vi "Read C.vi"(8 "error in (no error)":errorcluster, 11 "Arithemetic Operation in":refnum<class "Arithemetic Operation.lvclass">) -> (0 "error out":errorcluster, 2 "C":dbl, 3 "Arithemetic Operation out":refnum<class "Arithemetic Operation.lvclass">)   [LabVIEW 2023, in "Arithemetic Operation.lvclass"]
uses:
  Arithemetic Operation.lvclass
  Arithemetic Operation.lvclass/Arithemetic Operation.ctl
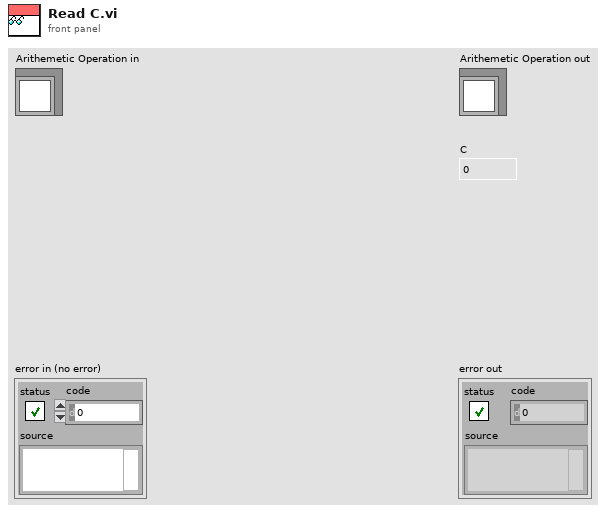
[diagram p1: front panel]
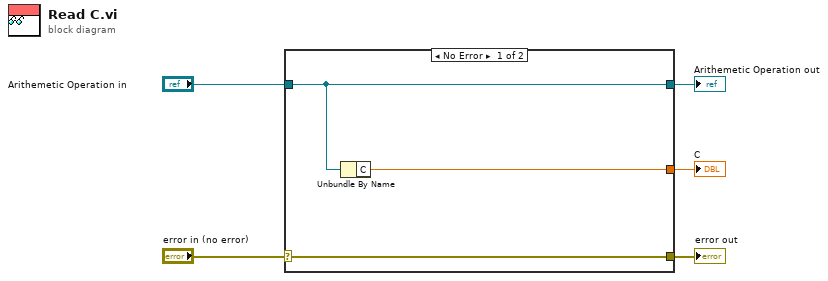
[diagram p0: block diagram]
diagram:
  n1 = case shown="No Error" "error in (no error)" {
    selector: "error in (no error)" -> [w8 w9]
    tunnel: [w8 w9] -> w4
    tunnel: [w7 w10] -> w2
    tunnel: "Arithemetic Operation in" -> [w7 w10]
    tunnel: [w6 _] -> w1
    frame No Error {
      n2 = Unbundle By Name(w7) -> ("C"=w6:dbl)
    }
    frame Error {
    }
  }
  "error out" <- w4
  "Arithemetic Operation out" <- w2
  "C" <- w1
